vi "Get Project Types.vi"(10 "Project:Active Project":refnum<vi>) -> (2 "Type Name Library File Path":map{string, map{string, path}}(c390))   [LabVIEW 2021, in "_Shared.lvlib"]
uses:
  _Shared.lvlib
  <vilib>/Nathan Davis/jettl/jettl/Queue/Queue.lvclass
  <vilib>/Nathan Davis/jettl/jettl/Event/Event.lvclass
  <vilib>/Nathan Davis/jettl/jettl/Msg Strategy/Msg Strategy.lvclass
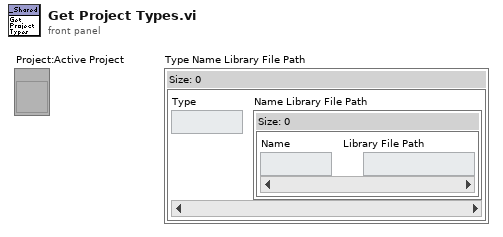
[diagram p1: front panel]
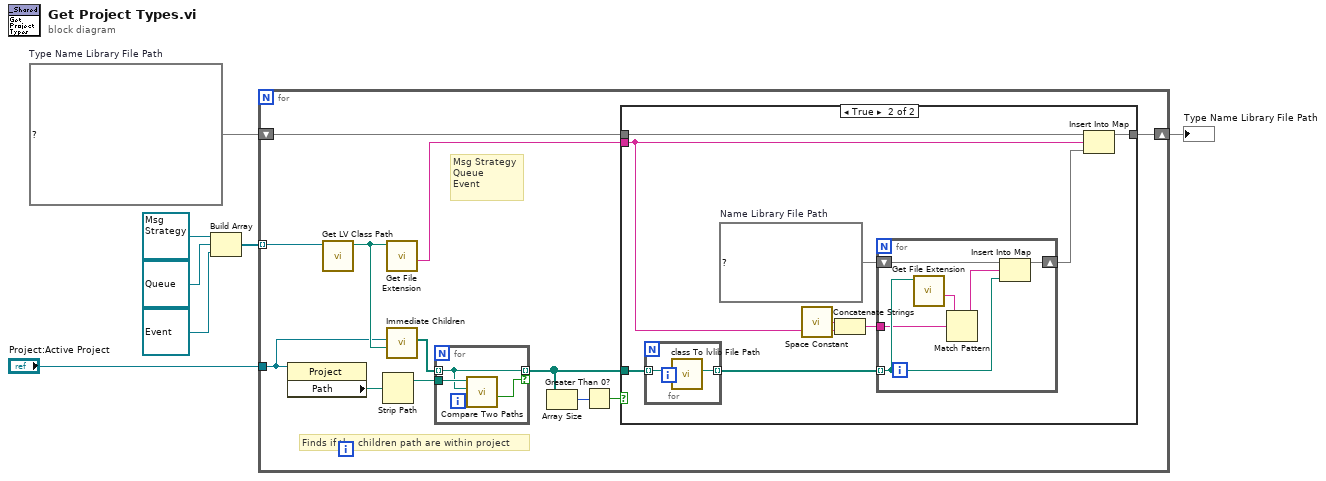
[diagram p0: block diagram]
diagram:
  w7 = map{string, map{string, path}} {}  # Type Name Library File Path
  n1 = Build Array(refnum<class "Msg Strategy.lvclass"> refnum ("jettl.lvlib:Msg Strategy.lvclass"), refnum<class "Queue.lvclass"> refnum ("jettl.lvlib:Queue.lvclass"), refnum<class "Event.lvclass"> refnum ("jettl.lvlib:Event.lvclass")) -> (w3:refnum<class>[])
  n2 = for {
    shift-right: [w14] -> w1
    shift-left: w7 -> [w15]
    tunnel: w3 -> [w13] mode=indexing
    tunnel: "Project:Active Project" -> [w8]
    # "Msg Strategy\nQueue\nEvent"
    # "Finds if the children path are within project"
    n3 = property class="Project"(reference=w8) -> ("Path"=w11:path)  [unwired: 1 in, 2 out]
    n4 = call <vilib>:"Get LV Class Path.vi"("object"=w13) -> ("class path"=w9:path)  [unwired: 9 in, 1 out]
    n5 = Strip Path(path=w11) -> (stripped path=w10:path)  [unwired: 1 out]
    n6 = call <vilib>:"Get File Extension.vi"("file"=w9) -> ("filename without extension"=w12:string)  [unwired: 6 in, 4 out]
    n7 = call "Immediate Children.vi"("Type File Path"=w9, "Project:Active Project"=w8) -> ("Implemented Class File Paths"=w19:path[])  [unwired: 8 in, 1 out]
    n8 = for {
      tunnel: w19 -> [w38] mode=indexing
      tunnel: [w38] -> w17 mode=indexing if=w40
      tunnel: w10 -> [w39]
      n9 = call <vilib>:"Compare Two Paths.vi"("Path 2"=w38, "Path 1"=w39) -> ("Path 2 Relative to Path 1?"=w40:bool)  [unwired: 6 in, 3 out]
    }
    n10 = Array Size(array=w17) -> (size(s)=w18:i32)
    n11 = Greater Than 0?(x=w18) -> (x > 0?=w16:bool)
    n12 = case shown="True" w16 {
      tunnel: w17 -> [_ w25]
      tunnel: w12 -> [_ w22]
      tunnel: w15 -> [w20 w29]
      tunnel: [w20 w28] -> w14
      frame False {
      }
      frame True {
        w26 = map{string, path} {}  # Name Library File Path
        n13 = for {
          tunnel: w25 -> [w31] mode=indexing
          tunnel: [w30] -> w24 mode=indexing
          n14 = call "class To lvlib File Path.vi"("Class File Path"=w31) -> ("Library File Path"=w30:path)  [unwired: 10 in]
        }
        n15 = call <vilib>:"Space Constant.vi"() -> ("String"=w23:string)
        n16 = Concatenate Strings(w23, w22) -> (w21:string)
        n17 = for {
          tunnel: w24 -> [w34] mode=indexing
          tunnel: w21 -> [w32]
          shift-right: [w36] -> w27
          shift-left: w26 -> [w37]
          n18 = call <vilib>:"Get File Extension.vi"("file"=w34) -> ("filename without extension"=w33:string)  [unwired: 6 in, 4 out]
          n19 = Match Pattern(string=w33, regular expression=w32) -> (before substring=w35:string)  [unwired: 1 in, 3 out]
          n20 = Insert Into Map(map in=w37, key=w35, value=w34) -> (map out=w36:map{string, path})  [unwired: 2 out]
        }
        n21 = Insert Into Map(map in=w29, key=w22, value=w27) -> (map out=w28:map{string, map{string, path}})  [unwired: 2 out]
      }
    }
  }
  "Type Name Library File Path" <- w1
